vi "fit_sos_st.vi"(0 "frf_data":T2, 7 "error in (no error)":errorcluster) -> (20 "theta":dbl[](array[numeric]), 22 "fit_sos_result":T1, 27 "error out":errorcluster)   [LabVIEW 2017]
doc: "DLL_PUBLIC int fit_sos_st(int N_omegas, double *omegas, double *resp_real,\n double *resp_imag, int N_theta, double *theta, mp_result *mpres)\n#endif\n\n\n\n\n#ifndef MPFIT_H\n#define MPFIT_H\n\n\n#ifdef __cplusplus\nextern \"C\" {\n#endif\n\n\n#define MPFIT_VERSION \"1.3\"\n\n\nstruct mp_par_struct {\n int fixed;\n\nDLL_PUBLIC int fit_sos_st(int N_omegas, double *omegas, double *resp_real,\n double *resp_imag, int N_theta, double *theta,\n struct FitSOSResult *fit_sos_result);"
uses:
  controls/SOS_frf_data.ctl
  fit_sos_results.ctl
  c-src/libfit_zpk32_lv/libfit_zpk32_lv.lvlib
  c-src/libfit_zpk32.dll
panel:
  out "function return":i32
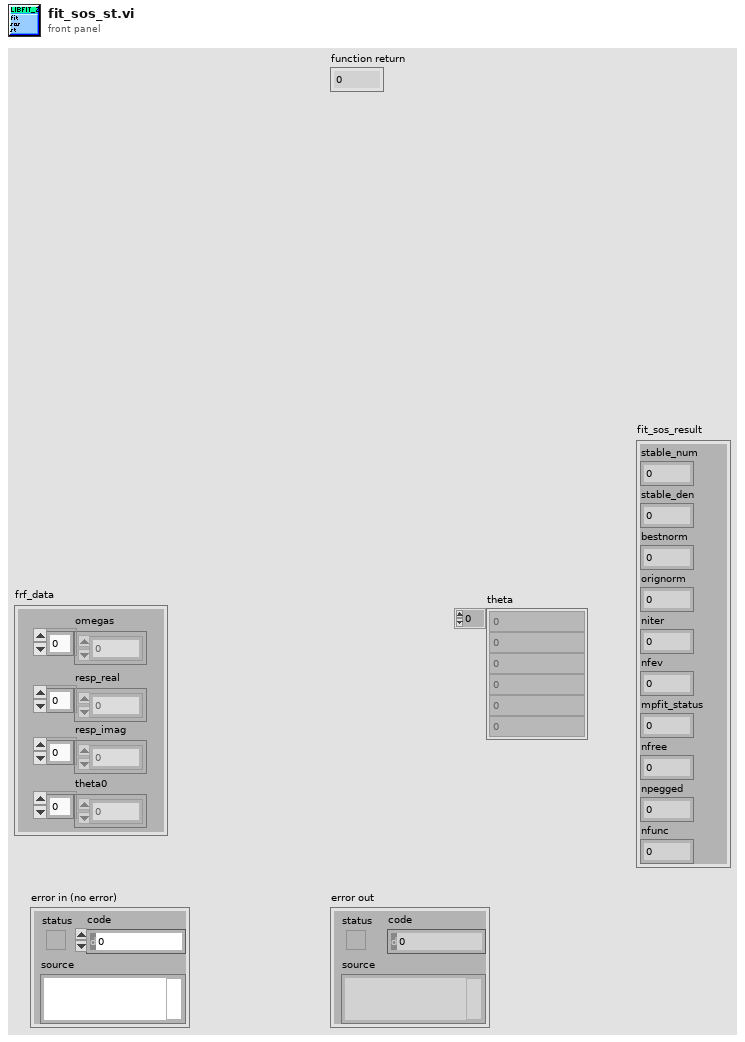
[diagram p1: front panel]
types:
  T1 = typedef "fit_sos_results.ctl" = cluster{"stable_num":i32, "stable_den":i32, "bestnorm":dbl, "orignorm":dbl, "niter":i32, "nfev":i32, "mpfit_status":i32, "nfree":i32, "npegged":i32, "nfunc":i32}
  T2 = typedef "SOS_frf_data.ctl" = cluster{"omegas":dbl[], "resp_real":dbl[], "resp_imag":dbl[], "theta0":dbl[]}
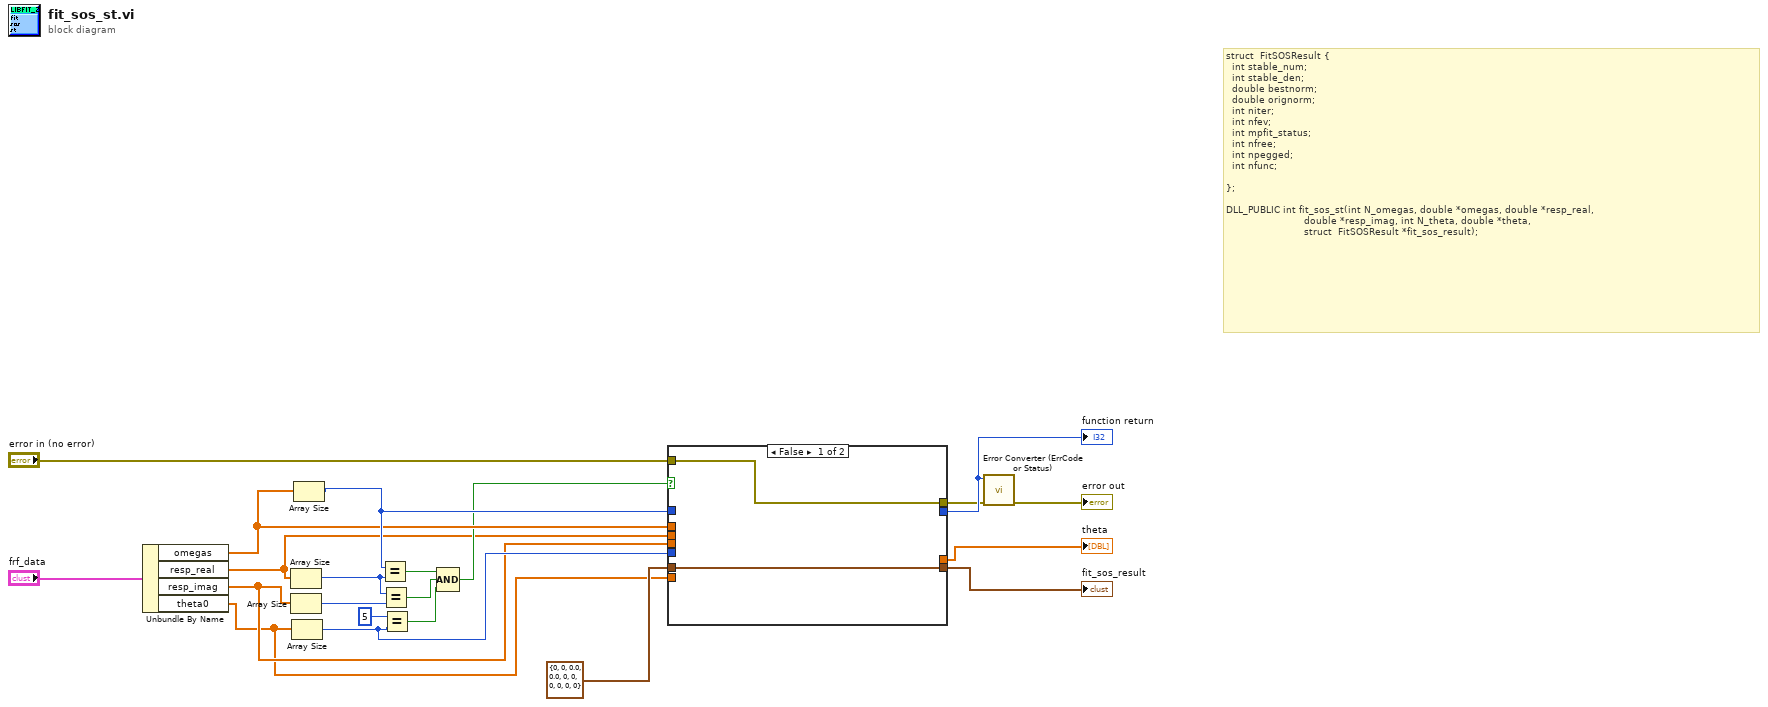
[diagram p0: block diagram]
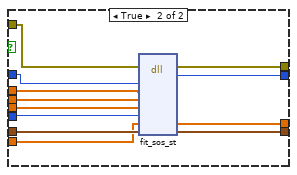
[diagram p2: hidden frame]
diagram:
  # "struct  FitSOSResult {\n  int stable_num;\n  int stable_den;\n  double bestnorm;\n  double orignorm;\n  int niter;\n  int nfev;\n  int mpfit_status;\n  int nfree;\n  int npegged;\n  int nfunc;\n\n};\n\nDLL_PUBLIC int fit_sos_st(int N_omegas, double *omegas, double *resp_real,\n                          double *resp_imag, int N_theta, double *theta,\n                          struct  FitSOSResult *fit_sos_result);"
  n1 = Unbundle By Name("frf_data") -> ("omegas"=w9:dbl[], "resp_real"=w7:dbl[], "resp_imag"=w5:dbl[], "theta0"=w4:dbl[])
  n2 = Array Size(array=w7) -> (size(s)=w14:i32)
  n3 = Array Size(array=w5) -> (size(s)=w15:i32)
  n4 = Array Size(array=w4) -> (size(s)=w6:i32)
  n5 = Array Size(array=w9) -> (size(s)=w10:i32)
  n6 = Equal?(x=w10, y=w14) -> (x = y?=w18:bool)
  n7 = Equal?(x=w14, y=w15) -> (x = y?=w17:bool)
  n8 = Equal?(x=5, y=w6) -> (x = y?=w12:bool)
  n9 = Compound Arithmetic op=AND(w18, w17, w12) -> (w8:bool)
  n10 = case shown="False" w8 {
    tunnel: [_ w35] -> w21
    tunnel: [_ w34] -> w2
    tunnel: [w22 w33] -> w1
    tunnel: [w23 w32] -> w20
    tunnel: T1 {"stable_num"=0, "stable_den"=0, "bestnorm"=0.0, "orignorm"=0.0, "niter"=0, "nfev"=0, "mpfit_status"=0, "nfree"=0, "npegged"=0, "nfunc"=0} ("fit_sos_result") -> [w22 w31]
    tunnel: w10 -> [_ w30]
    tunnel: w9 -> [_ w29]
    tunnel: w7 -> [_ w28]
    tunnel: w6 -> [_ w27]
    tunnel: w5 -> [_ w26]
    tunnel: w4 -> [_ w25]
    tunnel: "error in (no error)" -> [w23 w24]
    frame False {
    }
    frame True {
      n11 = dll-call lib="C:/Users/arnold/Documents/afm-cs/c-src/libfit_zpk32.*" fn="fit_sos_st"(error in=w24, "N_omegas"=w30, "omegas"=w29, "resp_real"=w28, "resp_imag"=w26, "N_theta"=w27, "theta"=w25, "fit_sos_result"=w31) -> (error out=w32:errorcluster, "return type"=w35:i32, "theta"=w34:dbl[], "fit_sos_result"=w33:T1)  [unwired: 7 in, 1 out]
    }
  }
  "function return" <- w21
  "theta" <- w2
  "fit_sos_result" <- w1
  n12 = call "Error Converter (ErrCode or Status).vi"("error in (no error)"=w20, "error code"=w21) -> ("error out"=→"error out":errorcluster)  [unwired: 9 in]
